vi "Elevator.vi"(0 "MotorControlDevRef":T1={"DeviceStatus"={"status"=FALSE, "code"=0, "source"=""}, "Type"=enum."PWM", "PWM"={"PWM Channel"=enum."Invalid", "DeadBand"={"Name"="", "maxPositivePwm"=0, "minPositivePwm"=0, "centerPwm"=0, "maxNegativePwm"=0, "minNegativePwm"=0, "angularRange"=0}}, "CAN"={"Device Number"=0, "Control Mode"=enum."Percent VBus", "Semaphore"=refnum, "Max Vout"=12.0, "TalonSRX Control Mode"=enum."Percent VBus"}, "Invert"=FALSE}, 2 "PID gains":T8={"proportional gain (Kc)"=1.0, "integral time (Ti, min)"=0.01, "derivative time (Td, min)"=0.0} {"derivative time (Td, min)" format="%.3f"; "integral time (Ti, min)" format="%.3f"; "proportional gain (Kc)" format="%.3f"}, 3 "Upper":bool, 4 "Manual":bool, 5 "Lower":bool, 6 "Upper Limit":dbl, 7 "Lower Limit":dbl, 8 "Distance":dbl, 11 "Override Pilot":bool, 17 "Override CoPilot":bool) -> (22 "Height":dbl)   [LabVIEW 2015]
uses:
  <vilib>/Rock Robotics/WPI/MotorControl/WPI_MotorControlDeviceRef.ctl
  <vilib>/Rock Robotics/WPI/MotorControl/WPI_MotorControlType.ctl
  <vilib>/Rock Robotics/SystemInterfaces/DIO/FPGA_DIOPWMChannel.ctl
  <vilib>/Rock Robotics/WPI/PWM/WPI_PWMDeadband.ctl
  <vilib>/Rock Robotics/WPI/CAN/Jaguar/SubVIs/WPI_CANJaguar_ControlMode.ctl
  <vilib>/Rock Robotics/WPI/CAN/TalonSRX/WPI_CANTalonSRX_APIControlMode.ctl
  <vilib>/addons/control/pid/pid.llb/PID (DBL).vi
  <vilib>/addons/control/pid/NI_PID_pid.lvlib
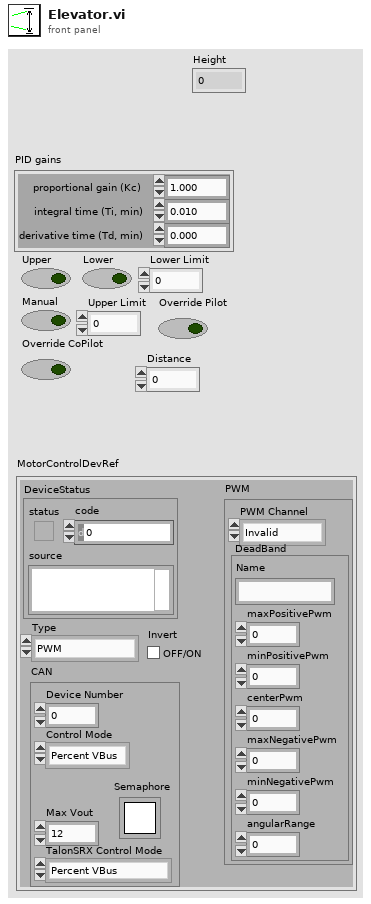
[diagram p1: front panel]
types:
  T1 = typedef "WPI_MotorControlDeviceRef.ctl" = cluster{"DeviceStatus":errorcluster, "Type":T2, "PWM":cluster{"PWM Channel":T3, "DeadBand":T4}, "CAN":cluster{"Device Number":u8, "Control Mode":T5, "Semaphore":T6, "Max Vout":dbl, "TalonSRX Control Mode":T7}, "Invert":bool}
  T2 = typedef "WPI_MotorControlType.ctl" = enum16{"PWM", "CAN", "CANTalonSRX"}
  T3 = typedef "FPGA_DIOPWMChannel.ctl" = enum8{"PWM 0", "PWM 1", "PWM 2", "PWM 3", "PWM 4", "PWM 5", "PWM 6", "PWM 7", "PWM 8", "PWM 9", "PWM MXP 0", "PWM MXP 1", "PWM MXP 2", "PWM MXP 3", "PWM MXP 4", "PWM MXP 5", "PWM MXP 6", "PWM MXP 7", "PWM MXP 8", "PWM MXP 9", "Invalid"}
  T4 = typedef "WPI_PWMDeadband.ctl" = cluster{"Name":string, "maxPositivePwm":i32, "minPositivePwm":i32, "centerPwm":i32, "maxNegativePwm":i32, "minNegativePwm":i32, "angularRange":u16}
  T5 = typedef "WPI_CANJaguar_ControlMode.ctl" = enum8{"Percent VBus", "Current", "Speed", "Position", "Voltage"}
  T6 = typedef "Semaphore RefNum" = refnum<k1>
  T7 = typedef "WPI_CANTalonSRX_APIControlMode.ctl" = enum8{"Percent VBus", "Speed", "Position", "Slave", "Unchanged / Invalid", "Voltage Compensation", "Current", "Motion Profile"}
  T8 = cluster{"proportional gain (Kc)":dbl, "integral time (Ti, min)":dbl, "derivative time (Td, min)":dbl}
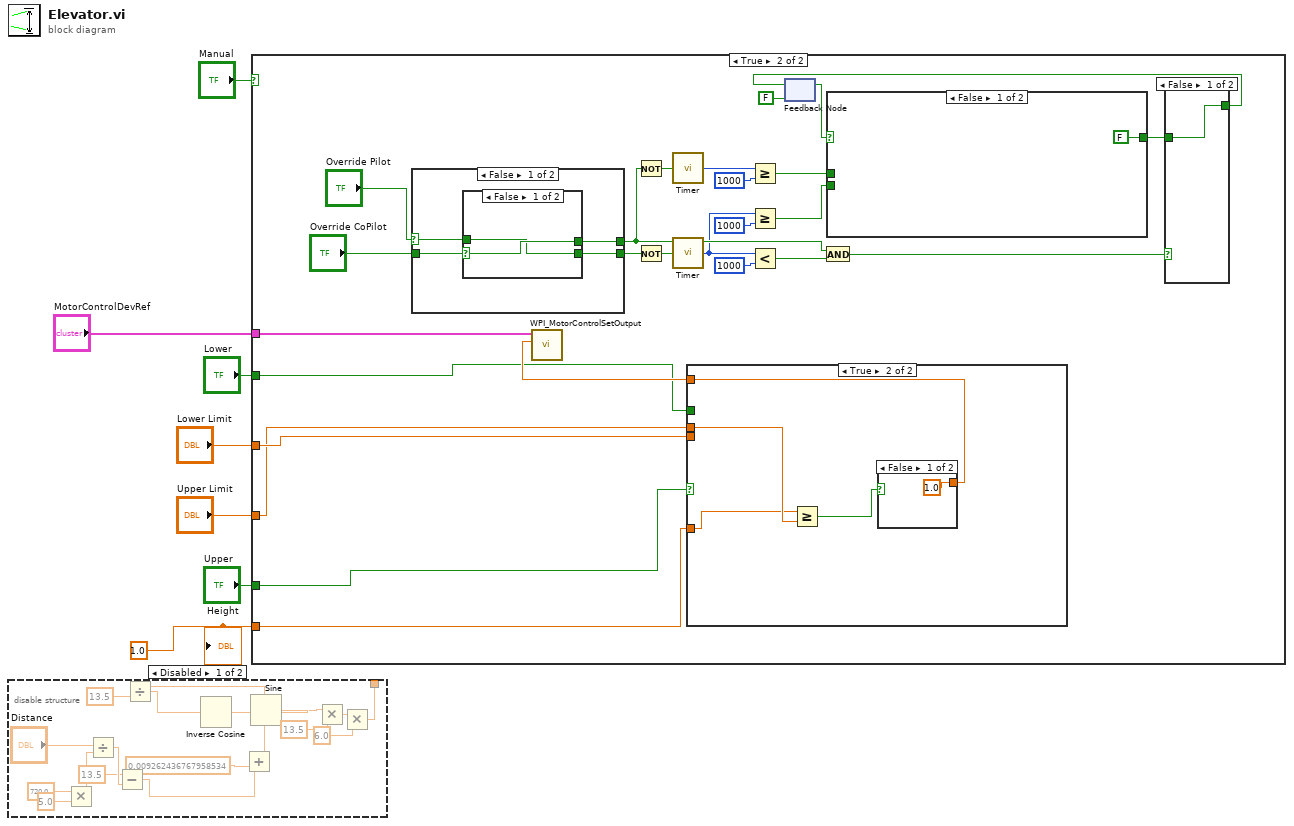
[diagram p0: block diagram]
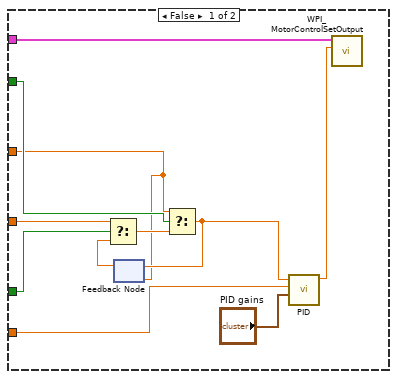
[diagram p3: hidden frame]
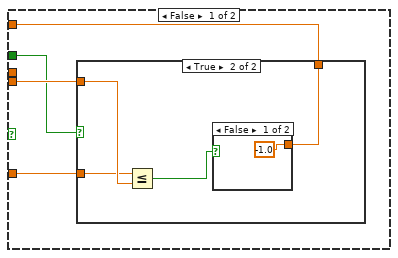
[diagram p4: hidden frame]
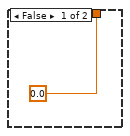
[diagram p5: hidden frame]
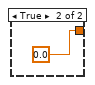
[diagram p6: hidden frame]
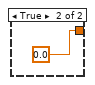
[diagram p7: hidden frame]
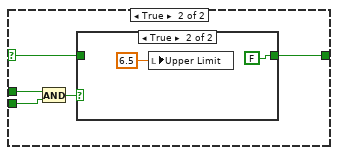
[diagram p8: hidden frame]
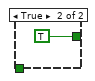
[diagram p10: hidden frame]
diagram:
  w1 = 1.0
  n1 = disable-structure shown="Disabled" {
    disable-tunnel: [w13 _] -> _
    frame Disabled {
      n2 = Multiply(x=720.0, y=5.0) -> (x*y=w23:dbl)
      n3 = Divide(x="Distance", y=w23) -> (x/y=w12:dbl)
      n4 = Subtract(x=13.5, y=w12) -> (x-y=w10:dbl)
      n5 = Add(x=w10, y=0.009262436767958534) -> (x+y=w9:dbl)
      n6 = Divide(x=w9, y=13.5) -> (x/y=w19:dbl)
      n7 = Inverse Cosine(1:w19) -> (0:w18:dbl)
      n8 = Sine(x=w18) -> (sin(x)=w17:dbl)
      n9 = Multiply(x=w17, y=13.5) -> (x*y=w15:dbl)
      n10 = Multiply(x=w15, y=6.0) -> (x*y=w13:dbl)
    }
    frame Enabled {
    }
  }
  n11 = case shown="True" "Manual" {
    tunnel: "Upper" -> [w31 w37]
    tunnel: "Lower" -> [w30 w38]
    tunnel: "MotorControlDevRef" -> [w28 w61]
    tunnel: "Upper Limit" -> [w27 w39]
    tunnel: "Lower Limit" -> [w25 w41]
    tunnel: w1 -> [w26 w36]
    frame False {
      n12 = feedback #1(w25) -> (w32:dbl)
      n13 = Select(t=w27, s=w31, f=w32) -> (s? t:f=w34:dbl)
      n14 = Select(t=w25, s=w30, f=w34) -> (s? t:f=w33:dbl)
      n15 = feedback-in #1(w33) -> ()
      n16 = call-poly <vilib>:"PID.vi"("PID gains"="PID gains", "process variable"=w26, "setpoint"=w33) -> ("output"=w29:dbl)  [unwired: 7 in, 1 out]
      n17 = call <vilib>:"WPI_MotorControlSetOutput.vi"("Output"=w29, "MotorControlDevRef"=w28) -> ()  [unwired: 7 in, 3 out]
    }
    frame True {
      n18 = case shown="False" "Override Pilot" {
        selector: "Override Pilot" -> [w90 w99]
        tunnel: "Override CoPilot" -> [w93 w98]
        tunnel: [w92 w98] -> w53
        tunnel: [w91 w99] -> w48
        frame False {
          n19 = case shown="False" w93 {
            selector: w93 -> [w95 w97]
            tunnel: [w95 w96] -> w92
            tunnel: [w94 w97] -> w91
            tunnel: w90 -> [w94 w96]
            frame False {
            }
            frame True {
            }
          }
        }
        frame True {
        }
      }
      n20 = Not(x=w53) -> (.not. x?=w51:bool)
      n21 = Not(x=w48) -> (.not. x?=w42:bool)
      n22 = call "Timer.vi"("Start Timer"=w51) -> ("Time elapsed"=w52:u64)
      n23 = call "Timer.vi"("Start Timer"=w42) -> ("Time elapsed"=w45:u64)
      n24 = case shown="True" w37 {
        tunnel: w41 -> [w65 _]
        tunnel: [w64 w74] -> w40
        tunnel: w39 -> [_ w75]
        tunnel: w38 -> [w63 _]
        tunnel: w36 -> [w62 w73]
        frame False {
          n25 = case shown="True" w63 {
            tunnel: w65 -> [_ w70]
            tunnel: [0.0 ("f") w68] -> w64
            tunnel: w62 -> [_ w67]
            frame False {
            }
            frame True {
              n26 = Less Or Equal?(x=w67, y=w70) -> (x <= y?=w69:bool)
              n27 = case shown="False" w69 {
                tunnel: [-1.0 ("f") 0.0 ("f")] -> w68
                frame False {
                }
                frame True {
                }
              }
            }
          }
        }
        frame True {
          n28 = Greater Or Equal?(x=w73, y=w75) -> (x >= y?=w76:bool)
          n29 = case shown="False" w76 {
            tunnel: [1.0 ("f") 0.0 ("f")] -> w74
            frame False {
            }
            frame True {
            }
          }
        }
      }
      n30 = call <vilib>:"WPI_MotorControlSetOutput.vi"("Output"=w40, "MotorControlDevRef"=w61) -> ()  [unwired: 7 in, 3 out]
      n31 = Greater Or Equal?(x=w52, y=u64 1000) -> (x >= y?=w58:bool)
      n32 = Greater Or Equal?(x=w45, y=u64 1000) -> (x >= y?=w57:bool)
      n33 = Less?(x=w45, y=u64 1000) -> (x < y?=w44:bool)
      n34 = feedback #2(FALSE) -> (w55:bool)
      n35 = And(x=w53, y=w44) -> (x .and. y?=w49:bool)
      n36 = case shown="False" w55 {
        selector: w55 -> [_ w80]
        tunnel: [FALSE w84] -> w56
        tunnel: w57 -> [_ w83]
        tunnel: w58 -> [_ w82]
        frame False {
        }
        frame True {
          n37 = And(x=w82, y=w83) -> (x .and. y?=w81:bool)
          n38 = case shown="True" w81 {
            tunnel: [w85 FALSE] -> w84
            tunnel: w80 -> [w85 _]
            frame False {
            }
            frame True {
              n39 = local write "Upper Limit"(6.5 ("Upper Limit")) -> ()
            }
          }
        }
      }
      n40 = case shown="False" w49 {
        tunnel: [w88 TRUE] -> w50
        tunnel: w56 -> [w88 _]
        frame False {
        }
        frame True {
        }
      }
      n41 = feedback-in #2(w50) -> ()
    }
  }
  "Height" <- w1
